vi "Port Number.vi"(0 "LV DEV.lvclass":refnum<class "LV DEV.lvclass">, 11 "Error In":errorcluster) -> (4 "LV DEV.lvclass":refnum<class "LV DEV.lvclass">, 6 "Machine name":string, 8 "Port Number":u16, 15 "error Out":errorcluster)   [LabVIEW 2019, in "LV DEV.lvclass"]
uses:
  LV DEV.lvclass
  <vilib>/regexp/Match Regular Expression.xnode
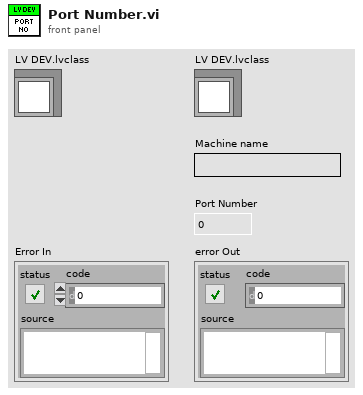
[diagram p1: front panel]
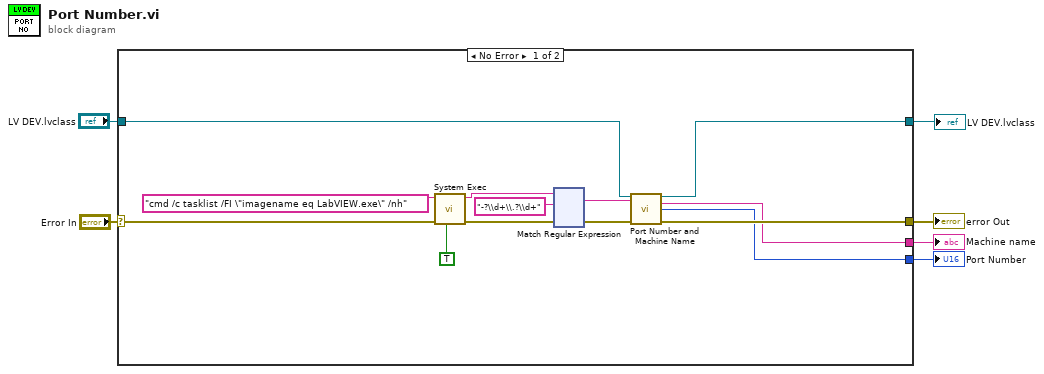
[diagram p0: block diagram]
diagram:
  n1 = case shown="No Error" "Error In" {
    selector: "Error In" -> [w19 w135]
    tunnel: [w13 w135] -> w5
    tunnel: "LV DEV.lvclass" -> [w9 w134]
    tunnel: [w8 w134] -> w1
    tunnel: [w12 _] -> w4
    tunnel: [w11 _] -> w3
    frame No Error {
      n2 = call <vilib>:"System Exec.vi"("run minimized? (F)"=TRUE, "error in (no error)"=w19, "command line"="cmd /c tasklist /FI \"imagename eq LabVIEW.exe\" /nh") -> ("error out"=w15:errorcluster, "standard output"=w17:string)  [unwired: 5 in, 2 out]
      n3 = xnode "Match Regular Expression"("input string"=w17, "regular expression"="-?\\d+\\.?\\d+", "error in"=w15) -> ("whole match"=w10:string, "error out"=w14:errorcluster)  [unwired: 3 in, 3 out]
      n4 = call "Port Number and Machine Name.vi"("LV DEV.lvclass"=w9, "PID"=w10, "error in (no error)"=w14) -> ("LV DEV.lvclass"=w8:refnum<class "LV DEV.lvclass">, "Machine Name"=w12:string, "Port Number"=w11:u16, "error out"=w13:errorcluster)  [unwired: 9 in]
    }
    frame Error {
    }
  }
  "error Out" <- w5
  "Port Number" <- w3
  "Machine name" <- w4
  "LV DEV.lvclass" <- w1
